vi "TxPkt - Update Properties.vi"(4 "Channel Data Types":string[](array[string]), 8 "error in (no error)":errorcluster, 9 "Channel Paths":string[](array[string]), 10 "Channel Names":string[](array[string]), 11 "Item Ref in":T1 format="%.0x") -> (0 "error out":errorcluster, 3 "Item Ref out":T1=18446744073709551615 format="%.0x")   [LabVIEW 2019, in "UDP-Custom-Device System Explorer.lvlib"]
uses:
  UDP-Custom-Device System Explorer.lvlib
  <vilib>/NI VeriStand/Custom Device API/Custom Device Item Ref.ctl
  <vilib>/NI VeriStand/Custom Device API/Custom Device API.lvlib
  Property Accessors/Tx Packet Accessors.lvlib
  Shared/UDP-Custom-Device Shared.lvlib
  Property Accessors/Shared Packet Accessors.lvlib
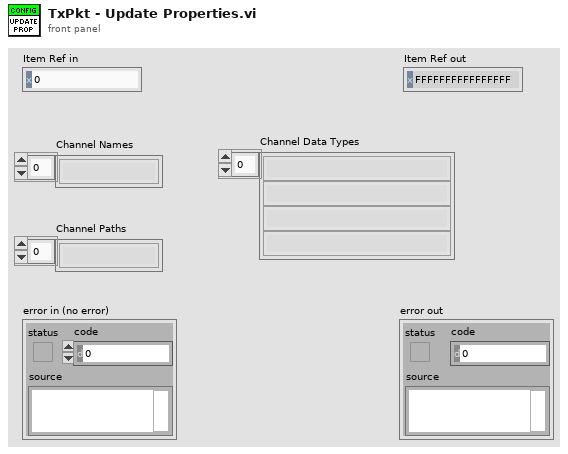
[diagram p1: front panel]
types:
  T1 = typedef "Custom Device API.lvlib/Custom Device Item Ref.ctl" = u64
  T2 = typedef "UDP-Custom-Device Shared.lvlib/Shared - Channel Data Type.ctl" = enum16{"Boolean", "Single", "Double", "I8", "I16", "I32", "I64", "U8", "U16", "U32", "U64"}
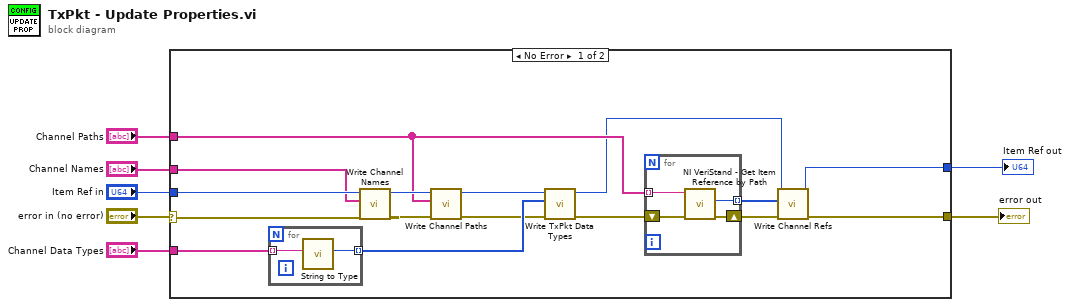
[diagram p0: block diagram]
diagram:
  n1 = case shown="No Error" "error in (no error)" {
    selector: "error in (no error)" -> [w19 w31]
    tunnel: [w9 w31] -> w7
    tunnel: "Item Ref in" -> [w20 w30]
    tunnel: [w8 w30] -> w5
    tunnel: "Channel Data Types" -> [w22 _]
    tunnel: "Channel Paths" -> [w15 _]
    tunnel: "Channel Names" -> [w18 _]
    frame No Error {
      n2 = for {
        tunnel: w22 -> [w25] mode=indexing
        tunnel: [w24] -> w21 mode=indexing
        n3 = call "String to Type.vi"("String Type"=w25) -> ("Data Type"=w24:T2)  [unwired: 10 in]
      }
      n4 = call "Write Channel Names.vi"("error in (no error)"=w19, "Channel Names"=w18, "Node Ptr"=w20) -> ("error out"=w14:errorcluster, "Node Ptr out"=w17:T1)  [unwired: 7 in]
      n5 = call "Write Channel Paths.vi"("error in (no error)"=w14, "Channel Paths"=w15, "Node Ptr"=w17) -> ("error out"=w13:errorcluster, "Node Ptr out"=w16:T1)  [unwired: 7 in]
      n6 = call "Write TxPkt Data Types.vi"("error in (no error)"=w13, "Data Types"=w21, "Node Ptr"=w16) -> ("error out"=w23:errorcluster, "Node Ptr out"=w12:T1)  [unwired: 7 in]
      n7 = for {
        shift-right: [w28] -> w10
        shift-left: w23 -> [w29]
        tunnel: w15 -> [w27] mode=indexing
        tunnel: [w26] -> w11 mode=indexing
        n8 = call <vilib>:"NI VeriStand - Get Item Reference by Path.vi"("error in (no error)"=w29, "Item Path in"=w27) -> ("error out"=w28:errorcluster, "Item Ref"=w26:T1)  [unwired: 6 in, 2 out]
      }
      n9 = call "Write Channel Refs.vi"("error in (no error)"=w10, "Dependent Node Refs"=w11, "Node Ptr"=w12) -> ("error out"=w9:errorcluster, "Node Ptr out"=w8:T1)  [unwired: 7 in]
    }
    frame Error {
    }
  }
  "error out" <- w7
  "Item Ref out" <- w5
